vi "ScaleInit.vi"(11 "VISA resource name":refnum<visa-resource-name>="COM11") -> (0 "error out":errorcluster, 3 "VISA Refnum out":refnum<visa-resource-name>)   [LabVIEW 2023]
uses:
  <vilib>/Instr/_visa.llb/VISA Configure Serial Port (Instr).vi
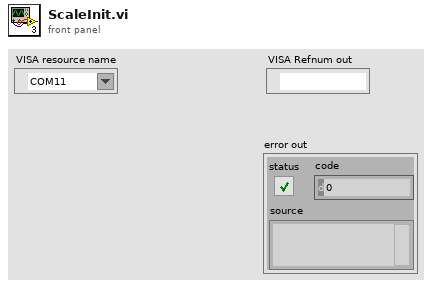
[diagram p1: front panel]
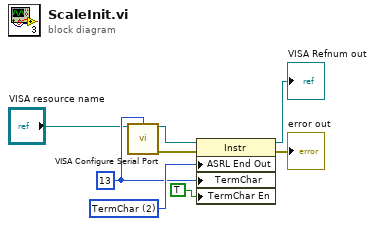
[diagram p0: block diagram]
diagram:
  w8 = u16 2 items=["None", "Last Bit", "TermChar", "Break"] ("Serial Settings:End Mode for Writes")
  w2 = u8 13 ("termination char\n(0xA = '\\n' = LF)")
  n1 = call-poly "VISA Configure Serial Port"("VISA resource name"="VISA resource name", "termination char\n(0xA = '\\n' = LF)"=w2) -> ("VISA resource name out"=w4:refnum<visa-resource-name>, "error out"=w5:errorcluster)  [unwired: 8 in, 4 out]
  n2 = property class="Instr"(reference=w4, error in=w5, "ASRL End Out"=w8, "TermChar"=w2, "TermChar En"=TRUE ("Message Based Settings:Termination Character Enable")) -> (reference out=→"VISA Refnum out":refnum<visa-resource-name>, error out=→"error out":errorcluster)
